vi "makeDecisions.vi"(8 "error in (no error)":errorcluster, 10 "model":refnum<class "Model.lvclass">, 11 "EnabledState in":refnum<class "WaitingForTestState.lvclass">) -> (0 "error out":errorcluster, 2 "model 2":refnum<class "Model.lvclass">, 3 "EnabledState out":refnum<class "WaitingForTestState.lvclass">)   [LabVIEW 2015, in "WaitingForTestState.lvclass"]
uses:
  WaitingForTestState.lvclass
  Model/Model/Model.lvclass
  Typedefs/StateSelector.ctl
  Typedefs/ILCBTTypedefs.lvlib
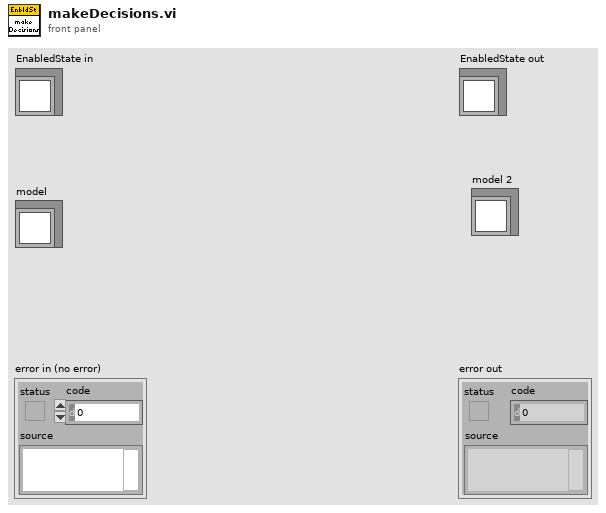
[diagram p1: front panel]
types:
  T1 = typedef "ILCBTTypedefs.lvlib/StateSelector.ctl" = enum16{"EnabledState", "FaultState", "OffState", "StandbyState"}
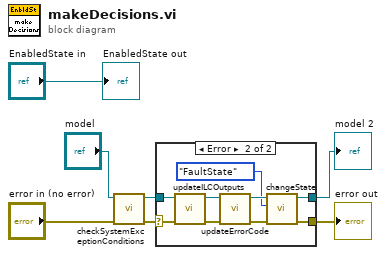
[diagram p0: block diagram]
diagram:
  n1 = call "checkSystemExceptionConditions.vi"("error in (no error)"="error in (no error)", "Model in"="model") -> ("error out"=w4:errorcluster, "Model out"=w3:refnum<class "Model.lvclass">)  [unwired: 8 in]
  n2 = case shown="Error" w4 {
    selector: w4 -> [w9 w12]
    tunnel: [w9 w16] -> w7
    tunnel: w3 -> [w8 w13]
    tunnel: [w8 w15] -> w5
    frame No Error {
    }
    frame Error {
      n3 = call "updateILCOutputs.vi"("error in (no error)"=w12, "Model in"=w13) -> ("error out"=w10:errorcluster, "Model out"=w11:refnum<class "Model.lvclass">)  [unwired: 8 in]
      n4 = call "updateErrorCode.vi"("error in (no error)"=w10, "Model in"=w11) -> ("error out"=w17:errorcluster, "Model out"=w18:refnum<class "Model.lvclass">)  [unwired: 8 in]
      n5 = call "changeState.vi"("error in (no error)"=w17, "State:"=StateSelector."FaultState", "Model in"=w18) -> ("error out"=w16:errorcluster, "Model out"=w15:refnum<class "Model.lvclass">)  [unwired: 7 in]
    }
  }
  "error out" <- w7
  "model 2" <- w5
  "EnabledState out" <- "EnabledState in"
